vi "PC_PumpMeas.vi"() -> ()   [LabVIEW 2020]
doc: "PC Controller Main VI"
uses:
  TypeDefs/ApplyMultiplier.ctl
  TypeDefs/NI9205offset.ctl
  TypeDefs/RTdisplayTimedLoop_dt.ctl
  TypeDefs/ApplyOffset.ctl
  TypeDefs/NI9205multiplier.ctl
  TypeDefs/NI9208offset.ctl
  TypeDefs/NI9208multiplier.ctl
  Components/DisplayWaveform/DisplayWaveforms/DisplayWaveforms.lvclass
  C:/Program Files (x86)/National Instruments/LabVIEW 2020/vi.lib/JKI/JKI SMO/SMO/SMO.lvclass
  C:/Program Files (x86)/National Instruments/LabVIEW 2020/vi.lib/JKI/JKI SMO/SMO.UI/SMO.UI.lvclass
  Components/DisplayWaveform/DisplayWaveforms/Typedefs/Dependencies--Cluster.ctl
  RT Target/PumpMeasurement/TypeDefs/STMLoopState_enum.ctl
  <vilib>/JKI/JKI SMO/SMO/Typedefs/SMOState --Enum.ctl
  Components_global/Queues/InterProcessQueueCtl.ctl
  TypeDefs/ConfigCluster.ctl
  TypeDefs/GraphInfoCluster.ctl
  <vilib>/NI/STM/TCP/TCP Read Options.ctl
  TypeDefs/AIloopTimes.ctl
  <vilib>/NI/STM/TCP/Read Meta Data (TCP Ref).vi
  f38d6d6a-e512-492a-acdc-1d388213210b.vi
  78bd2656-12e6-4809-88cd-6a89556620fb.vi
  <vilib>/NI/STM/TCP/Get Connection Reference (TCP).vi
  <vilib>/NI/STM/TCP/Read Meta Data (TCP Clst).vi
  <vilib>/JDP Science/JSONtext/JSON text to Variant.vi
  <vilib>/JDP Science/JSONtext/Variant to JSON Text.vi
  <vilib>/NI/STM/TCP/Read Message (TCP).vi
  <vilib>/NI/STM/TCP/Write Message (TCP).vi
  <vilib>/JDP Science/JSONtext/LVClass Serializer/JSONtext LVClass Serializer.lvclass
  <vilib>/NI/STM/NI STM.lvlib
  <vilib>/JKI/JKI SMO/SMO/SMO.lvclass
  <vilib>/JKI/JKI SMO/SMO.UI/SMO.UI.lvclass
  Components_global/Queues/Queues.lvlib
  <vilib>/JDP Science/JSONtext/JSONtext.lvlib
panel:
  in  "Update Chart?":bool
  in  "Clear Chart":bool
  in  "Export":bool
  in  "Stop":bool
  out "Status":string
  in  "Tab Control":enum32{"Information"}(tab)
  in  "NI9208 Multiplier":T1
  in  "NI9208 Offset":T2={"NI9208 Offset"=[0.0, 0.0, 0.0, 0.0, 0.0]}
  in  "NI9205 Multiplier":T3
  in  "Apply Offset?":T4
  out "NI9208 loop time [ms]":dbl=10.0 caption="Numeric"
  in  "RT Display Reader Loop Time [ms]":T5=1000 caption="Numeric"
  in  "Load\nConfig":bool
  in  "Save\nConfig":bool
  in  "NI9205 Offset":T6={"NI9205 Offset"=[0.0, 0.0, 0.0, 0.0, 0.0, 0.0, 0.0, 0.0, 0.0, 0.0, 0.0, 0.0, 0.0, 0.0, 0.0]}
  out "# of display elements \nunpacked (row x col)":i32[](array[numeric]) caption="Numeric"
  out "NI9205 loop time [ms]":dbl caption="Numeric"
  in  "Apply Multiplier?":T7
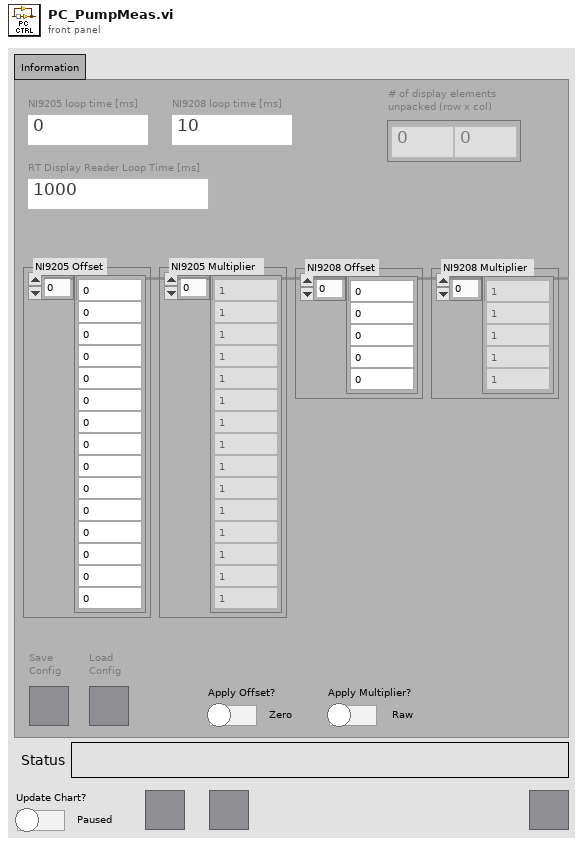
[diagram p1: front panel]
types:
  T1 = typedef "NI9208multiplier.ctl" = cluster{"NI9208 Multiplier":dbl[]}
  T2 = typedef "NI9208offset.ctl" = cluster{"NI9208 Offset":dbl[]}
  T3 = typedef "NI9205multiplier.ctl" = cluster{"NI9205 Multiplier":dbl[]}
  T4 = typedef "ApplyOffset.ctl" = bool
  T5 = typedef "RTdisplayTimedLoop_dt.ctl" = i64
  T6 = typedef "NI9205offset.ctl" = cluster{"NI9205 Offset":dbl[]}
  T7 = typedef "ApplyMultiplier.ctl" = bool
  T8 = typedef "STMLoopState_enum.ctl" = enum16{"Initialize", "Warm-up", "Run", "ShutDown"}
  T9 = typedef "DisplayWaveform.lvlib/DisplayWaveforms.lvclass/Dependencies--Cluster.ctl" = cluster{"New Value":refnum<user-event>}
  T10 = typedef "SMO.lvclass/Public Events.ctl" = cluster{"Error":refnum<user-event>, "State":refnum<user-event>, "Reserve State":refnum<user-event>}
  T11 = typedef "SMO.UI.lvclass/PublicEvents--Cluster.ctl" = cluster{"UI Hidden":refnum<user-event>, "UI State":refnum<user-event>}
  T12 = typedef "DisplayWaveform.lvlib/DisplayWaveforms.lvclass/PublicEvents--Cluster.ctl" = cluster{"Chart Cleared":refnum<user-event>, "Chart Exported":refnum<user-event>, "ChartParams Set":refnum<user-event>}
  T13 = typedef "NI STM.lvlib/TCP Connection Info.ctl" = cluster{"connection ID":refnum<k5>, "meta data":T14[]}
  T14 = typedef "NI STM.lvlib/MetaDataElement.ctl" = string
  T15 = typedef "Queues.lvlib/Queue Refs.ctl" = cluster{"InterProcessQueue":refnum<queue>}
  T16 = typedef "SMO.lvclass/SMOState --Enum.ctl" = enum16{"unknown", "Created", "Started", "Stopped"}
  T17 = enum32{"Invalid", "Standard", "Closed", "Hidden", "Minimized", "Maximized"}
  T18 = enum32{"invalid app kind", "Development System", "Run Time System", "Student Edition", "Embedded LabVIEW", "Evaluation", "Custom"}
  T19 = typedef "Queues.lvlib/InterProcessQueueCtl.ctl" = cluster{"Command":string, "Data":variant}
  T20 = typedef "ConfigCluster.ctl" = cluster{"RT Display Reader Loop Time [ms]":i64, "NI9205 Offset":T6, "NI9205 Multiplier":T3, "NI9208 Offset":T2, "NI9208 Multiplier":T1, "Apply Offset?":T4, "Apply Multiplier?":T7}
  T21 = enum16{"open", "replace", "create", "open or create", "replace or create", "replace or create with confirmation"}
  T22 = typedef "GraphInfoCluster.ctl" = cluster{"RT Display Reader Loop Time [ms]":T5, "NI9205 Offset":T6, "NI9205 Multiplier":T3, "NI9208 Offset":T2, "NI9208 Multiplier":T1}
  T23 = cluster{"Core":cluster{"Current VI Reference":refnum<vi>, "Close Panel on Exit?":bool}, "UI switch state":bool, "Export Folder Path":path}
  T24 = cluster{"Current VI Reference":refnum<vi>, "Close Panel on Exit?":bool}
  T25 = typedef "ChartParamsCluster.ctl" = cluster{"Chart ScaleMultipliers":cluster{"WF Xscale Multiplier":dbl, "WF Yscale Multiplier":dbl[]}, "NI9205 Offset":T6, "NI9205 Multipliers":T3, "NI9208 Offset":T2, "NI9208 Multiplier":T1}
  T26 = typedef "NI STM.lvlib/TCP Read Options.ctl" = cluster{"ignore timeout error":bool, "timeout ms (1000)":i32}
  T27 = typedef "AIloopTimes.ctl" = cluster{"NI 9205 loop time":dbl, "NI 9208 loop time":dbl}
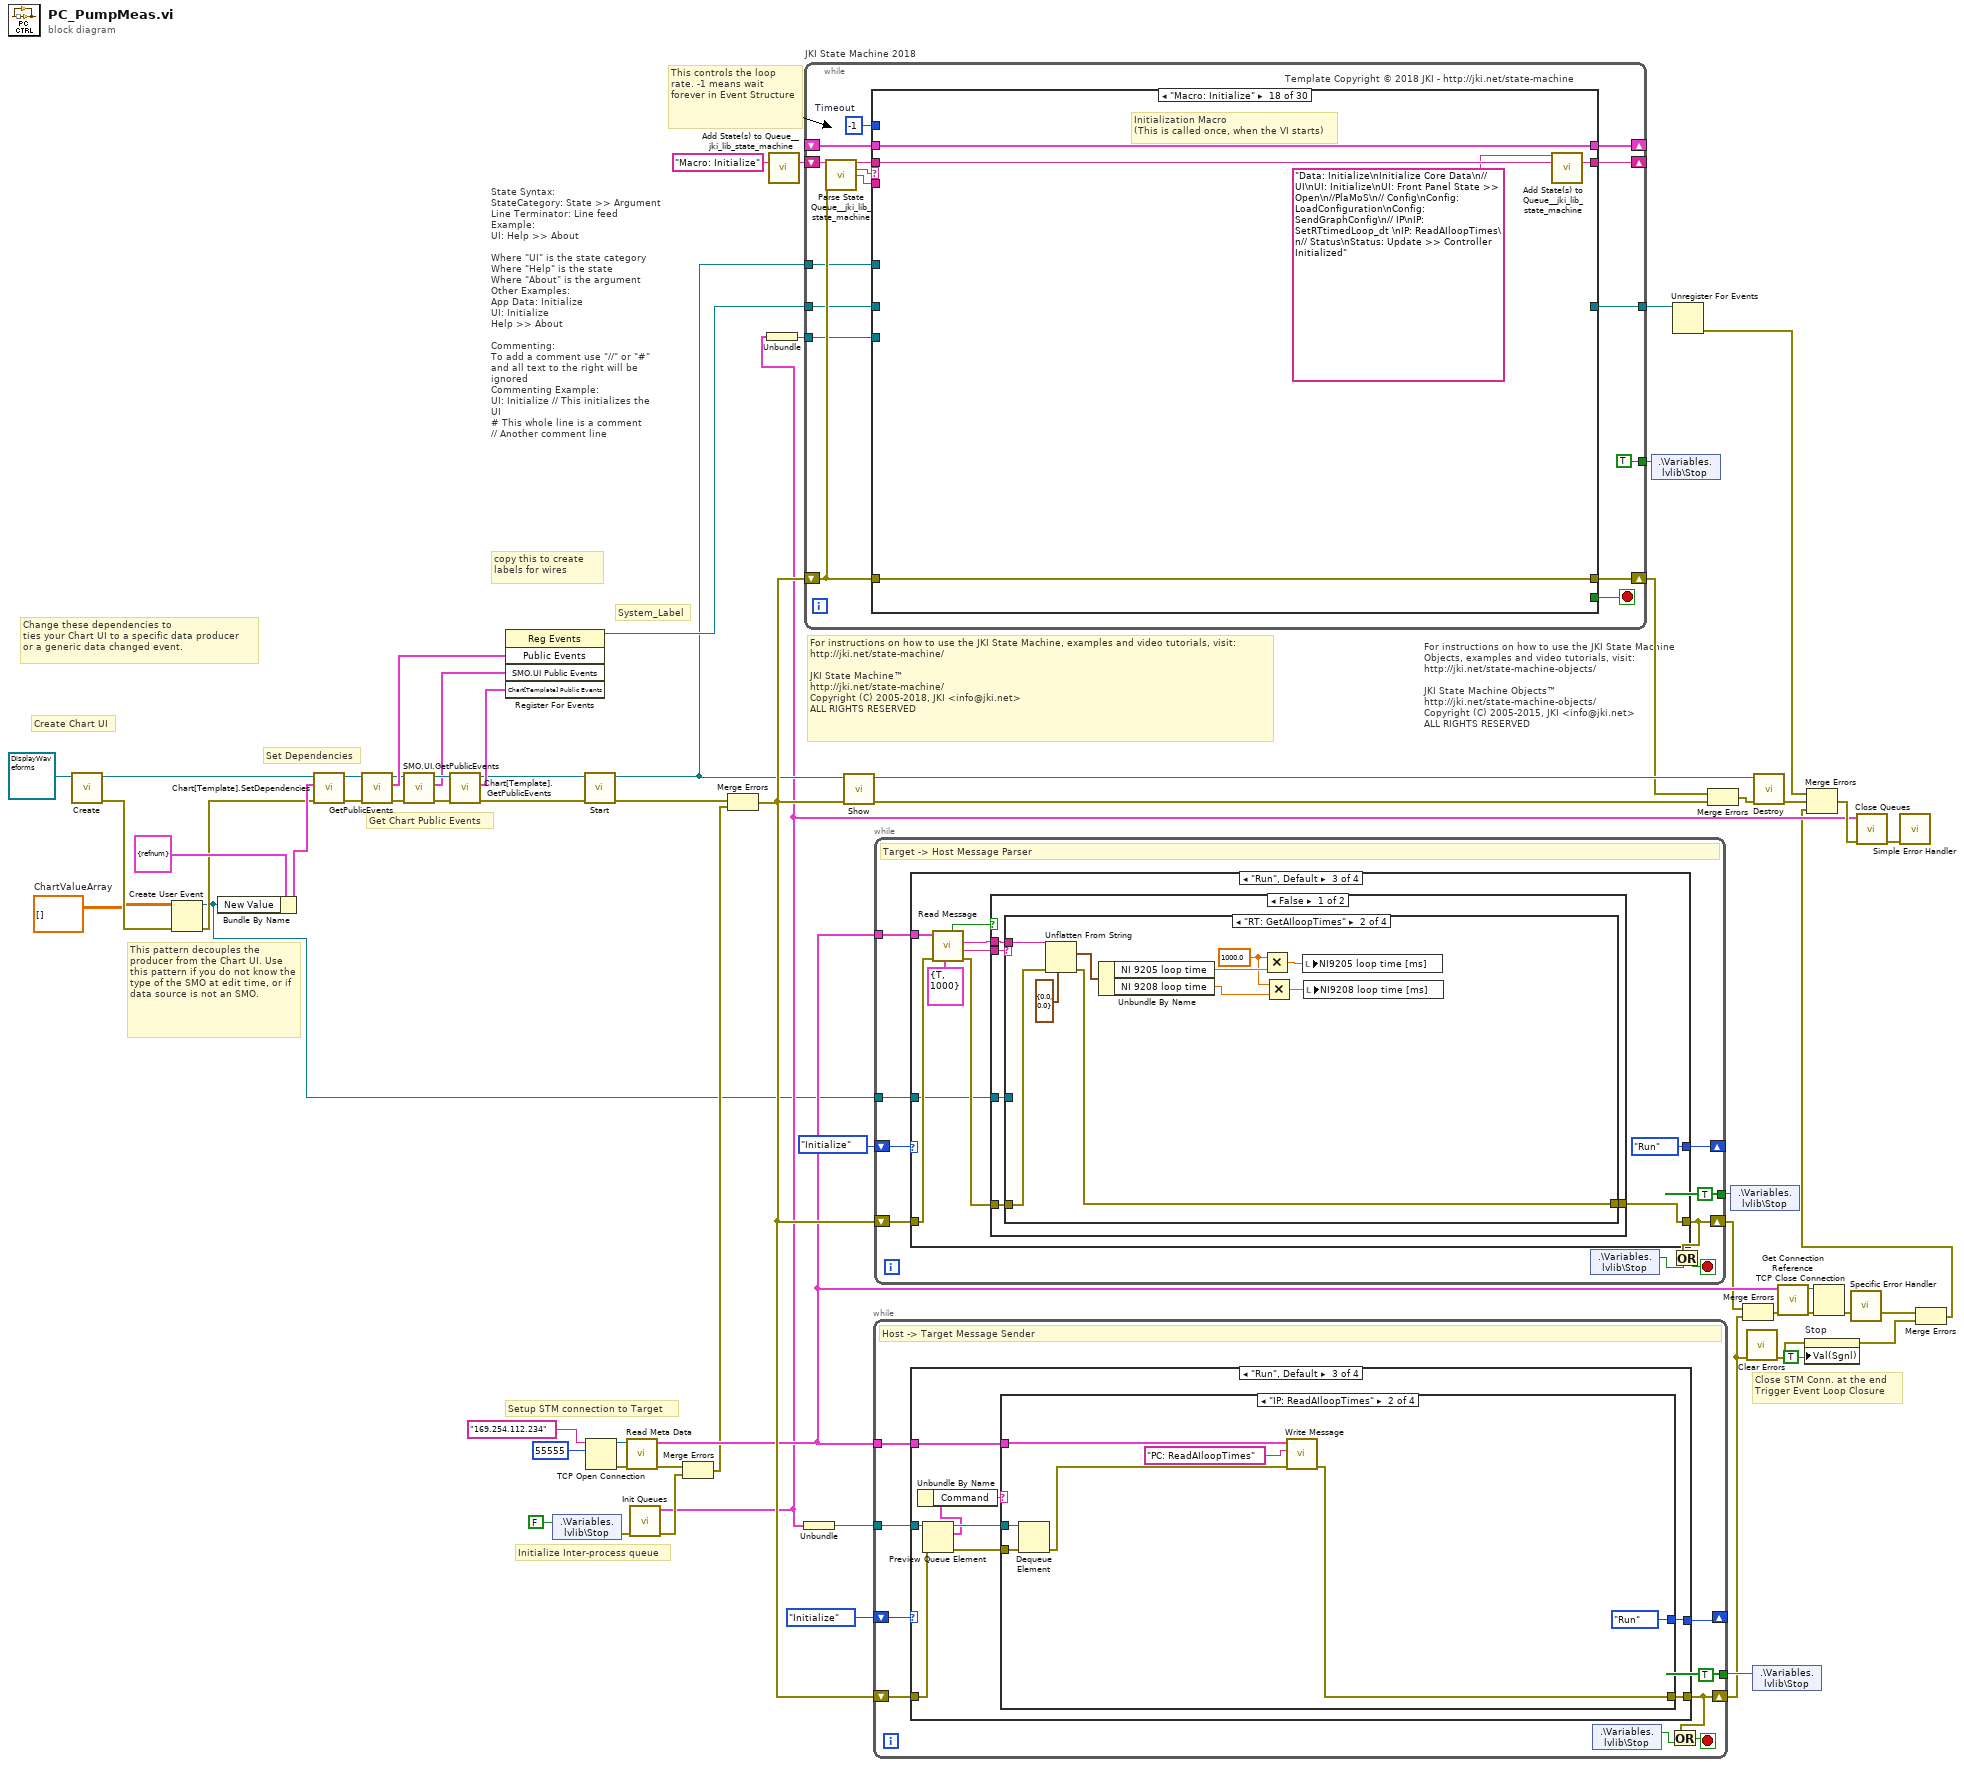
[diagram p0: block diagram]
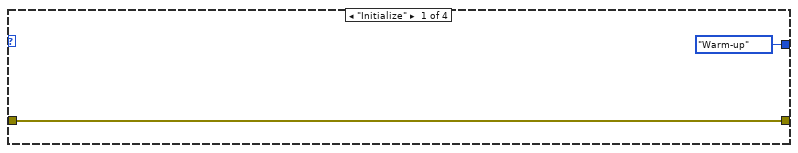
[diagram p2: hidden frame]
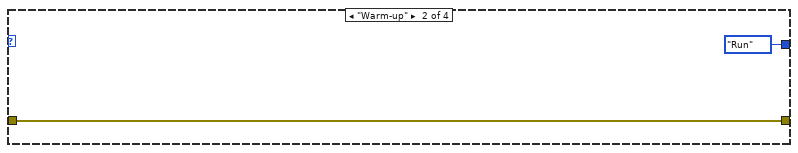
[diagram p3: hidden frame]
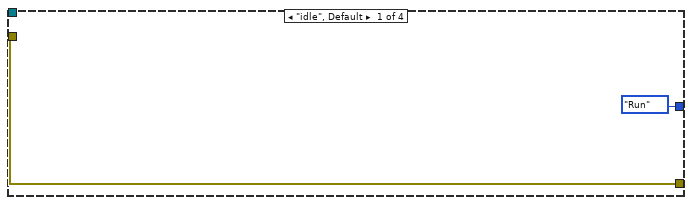
[diagram p4: hidden frame]
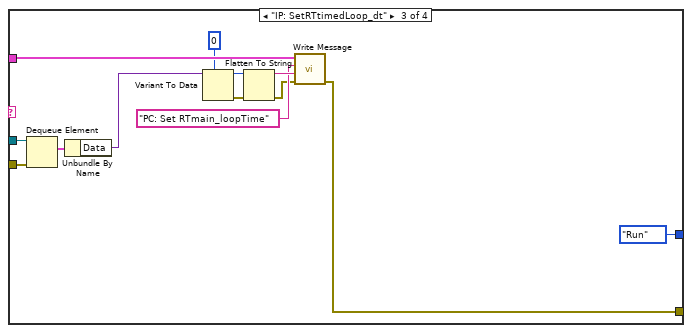
[diagram p5: hidden frame]
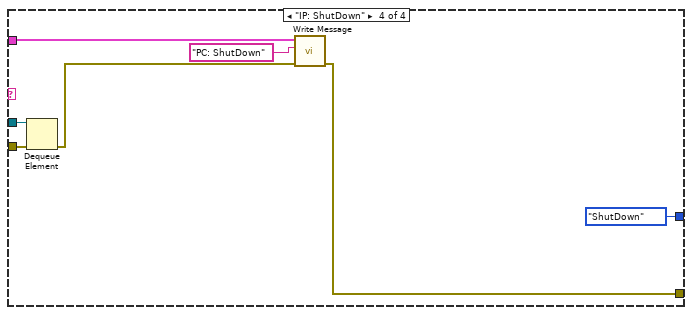
[diagram p6: hidden frame]
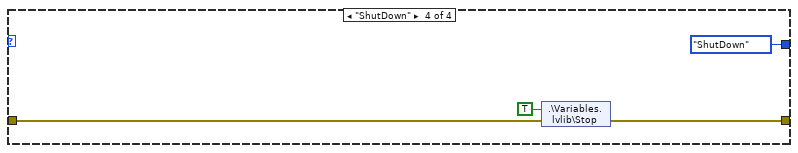
[diagram p7: hidden frame]
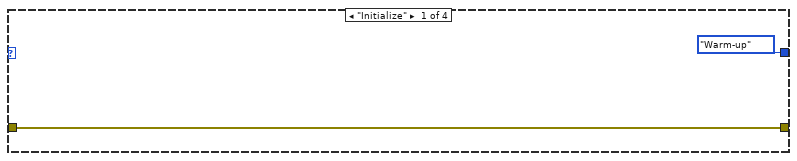
[diagram p8: hidden frame]
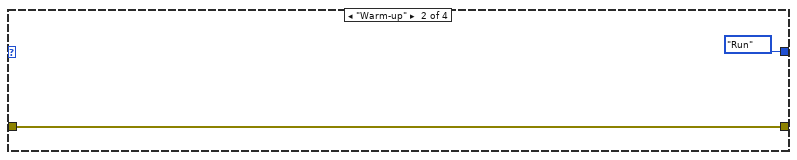
[diagram p9: hidden frame]
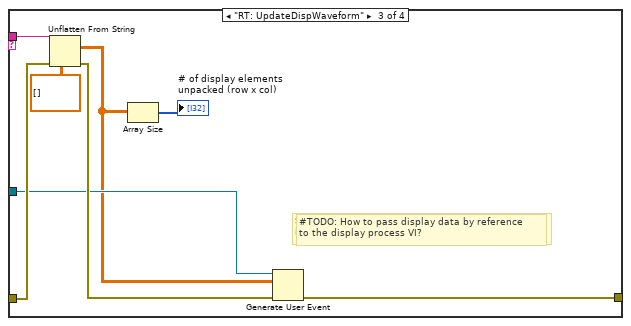
[diagram p11: hidden frame]
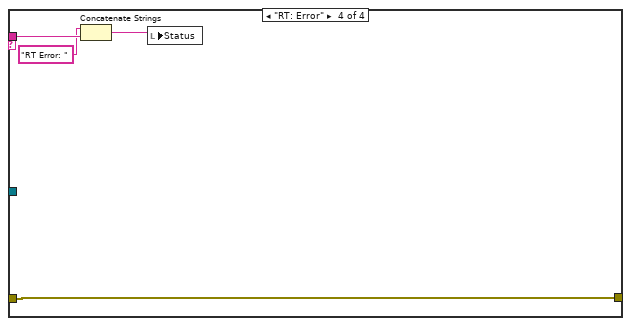
[diagram p12: hidden frame]
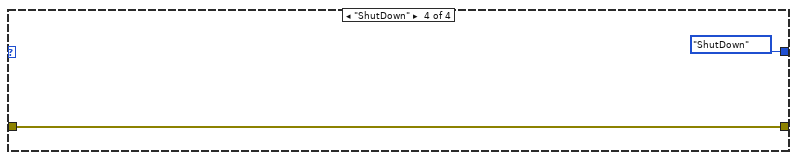
[diagram p14: hidden frame]
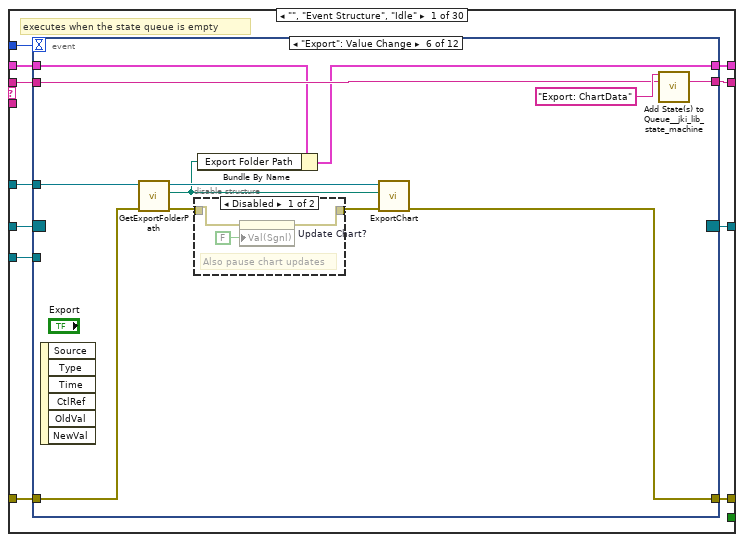
[diagram p15: hidden frame]
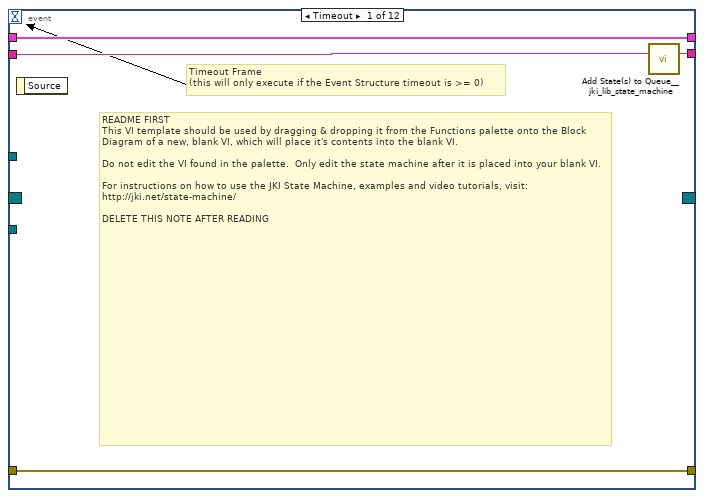
[diagram p16: hidden frame]
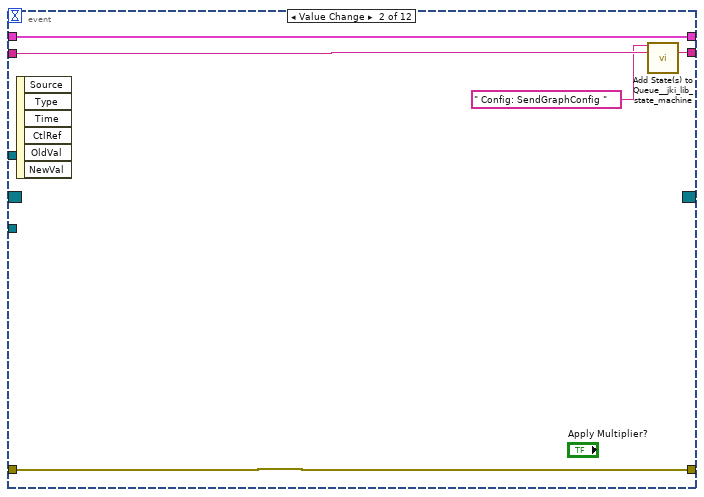
[diagram p17: hidden frame]
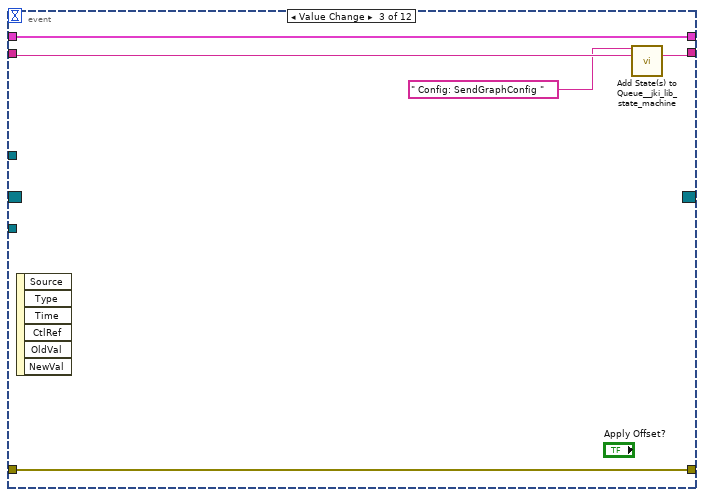
[diagram p18: hidden frame]
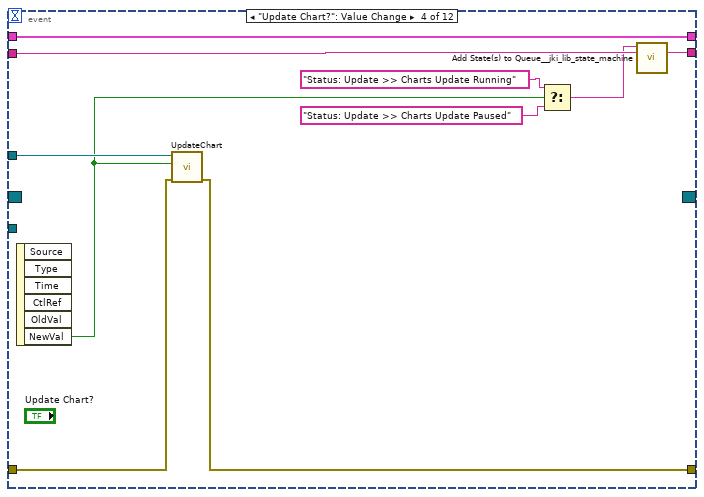
[diagram p19: hidden frame]
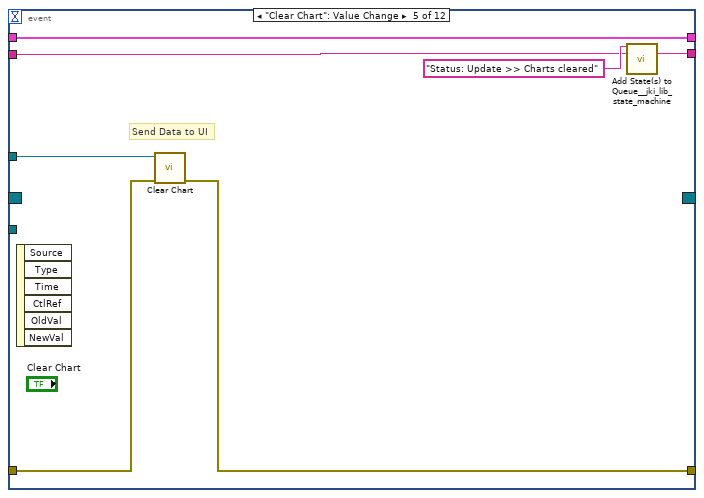
[diagram p20: hidden frame]
diagram:
  w9 = dbl[][] []  # ChartValueArray
  # "Close STM Conn. at the end\nTrigger Event Loop Closure"
  # "Setup STM connection to Target"
  # "Initialize Inter-process queue"
  # "This pattern decouples the producer from the Chart UI. Use this pattern if you do not know the type of the SMO at edit time, or if data source is not an SMO."
  # "For instructions on how to use the JKI State Machine, examples and video tutorials, visit:\nhttp://jki.net/state-machine/\n\nJKI State Machine™\nhttp://jki.net/state-machine/\nCopyright (C) 2005-2018, JKI <info@jki.net>\nALL RIGHTS RESERVED"
  # "State Syntax:\nStateCategory: State >> Argument\nLine Terminator: Line feed\nExample:\nUI: Help >> About\n\nWhere \"UI\" is the state category\nWhere \"Help\" is the state\nWhere \"About\" is the argument\nOther Examples:\nApp Data: Initialize\nUI: Initialize\nHelp >> About\n\nCommenting:\nTo add a comment use \"//\" or \"#\" and all text to the right will be ignored\nCommenting Example:\nUI: Initialize // This initializes the UI\n# This whole line is a comment\n// Another comment line"
  # "copy this to create labels for wires"
  # "This controls the loop rate. -1 means wait forever in Event Structure"
  # "System_Label"
  # "Set Dependencies"
  # "Create Chart UI"
  # "Change these dependencies to\nties your Chart UI to a specific data producer\nor a generic data changed event."
  # "For instructions on how to use the JKI State Machine Objects, examples and video tutorials, visit:\nhttp://jki.net/state-machine-objects/\n\nJKI State Machine Objects™\nhttp://jki.net/state-machine-objects/\nCopyright (C) 2005-2015, JKI <info@jki.net>\nALL RIGHTS RESERVED"
  # "Get Chart Public Events"
  n1 = call <vilib>:"Create.vi"("SMO"=refnum<class "DisplayWaveforms.lvclass"> refnum ("Chart[Template]")) -> ("error out"=w11:errorcluster, "SMO out"=w55:refnum<class "DisplayWaveforms.lvclass">)  [unwired: 8 in, 1 out]
  n2 = Create User Event(user event datatype=w9, error in=w11) -> (user event=w8:refnum<user-event>, error out=w10:errorcluster)
  n3 = Bundle By Name(cluster=T9 {"New Value"=refnum} ("Dependencies"), "New Value"=w8) -> (w53:T9)
  n4 = call "Chart[Template].SetDependencies.vi"("error in (no error)"=w10, "Dependencies"=w53, "DisplayWaveforms"=w55) -> ("error out"=w41:errorcluster, "DisplayWaveforms out"=w52:refnum<class "DisplayWaveforms.lvclass">)  [unwired: 7 in]
  n5 = call <vilib>:"GetPublicEvents.vi"("error in (no error)"=w41, "SMO"=w52) -> ("error out"=w47:errorcluster, "Public Events"=w51:T10, "SMO out"=w49:refnum<class "DisplayWaveforms.lvclass">)  [unwired: 7 in]
  n6 = call <vilib>:"SMO.UI.GetPublicEvents.vi"("error in (no error)"=w47, "SMO.UI"=w49) -> ("error out"=w46:errorcluster, "SMO.UI Public Events"=w45:T11, "SMO.UI out"=w48:refnum<class "DisplayWaveforms.lvclass">)  [unwired: 7 in]
  n7 = call "Chart[Template].GetPublicEvents.vi"("error in (no error)"=w46, "DisplayWaveforms"=w48) -> ("error out"=w42:errorcluster, "Chart[Template] Public Events"=w50:T12, "DisplayWaveforms out"=w43:refnum<class "DisplayWaveforms.lvclass">)  [unwired: 7 in]
  n8 = register-events(w51, w45, w50) -> (reference out=w44:refnum<event-registration>)  [unwired: 2 in, 1 out]
  n9 = shared-variable ".\\Variables.lvlib\\Stop"(FALSE ("Stop")) -> (error out=w32:errorcluster)  [unwired: 1 in]
  n10 = call <vilib>:"Start.vi"("error in (no error)"=w42, "SMO"=w43) -> ("error out"=w27:errorcluster, "SMO out"=w25:refnum<class "DisplayWaveforms.lvclass">)  [unwired: 8 in]
  n11 = TCP Open Connection(address="169.254.112.234" ("Target IP Address"), remote port or service name=u16 55555 ("remote port")) -> (connection ID=w63:refnum<k5>, error out=w62:errorcluster)  [unwired: 1 in, 2 out]
  n12 = call-poly <vilib>:"Read Meta Data.vi"("error in"=w62, "connection ID"=w63) -> ("error out"=w16:errorcluster, "connection info out"=w21:T13)  [unwired: 1 in, 7 out]
  n13 = call "Init Queues.vi"("error in (no error)"=w32) -> ("error out"=w15:errorcluster, "Queue Refs"=w12:T15)  [unwired: 9 in]
  n14 = Merge Errors(w16, w15) -> (w14:errorcluster)
  n15 = Merge Errors(w27, w14) -> (w26:errorcluster)
  n16 = Unbundle(w12) -> ("InterProcessQueue"=w13:refnum<queue>)
  n17 = call <vilib>:"Add State(s) to Queue__jki_lib_state_machine.vi"("State(s) in (\"\")"="Macro: Initialize") -> ("States Out"=w39:string)  [unwired: 14 in]
  n18 = Unbundle(w12) -> ("InterProcessQueue"=w28:refnum<queue>)
  n19 = while "JKI State Machine 2018" {
    shift-right: [w66] -> _
    shift-left: _ -> [w72]
    shift-right: [w74] -> _
    shift-left: w39 -> [w76]
    tunnel: w44 -> [w69]
    tunnel: w25 -> [w68]
    tunnel: [w67] -> w37
    tunnel: [TRUE ("Stop")] -> w35
    shift-right: [w75] -> w7
    shift-left: w26 -> [w70]
    tunnel: w13 -> [w64]
    stop <- w73 stop-if-true
    w71 = -1  # Timeout
    # "Template Copyright © 2018 JKI - http://jki.net/state-machine"
    n20 = call <vilib>:"Parse State Queue__jki_lib_state_machine.vi"("State Queue"=w76, "Error In (no error)"=w70) -> ("Remaining States"=w78:string, "Current State"=w79:string, "Arguments"=w77:string)  [unwired: 11 in]
    n21 = case shown="\"Macro: Initialize\"" w79 {
      selector: w79 -> [_ _ w188 _ _ _ _ _ _ _ _ _ _ _ _ _ _ _ _ _ _ _ _ _ _ _ _ _ _ _]
      tunnel: w78 -> [w90 w187 w192 w211 w213 w225 w229 w236 w242 w246 w254 w263 w274 w343 w352 w364 w368 w373 w390 w394 w423 w451 w474 w493 w502 w506 w511 w515 w519 w523]
      tunnel: w77 -> [_ _ _ _ _ _ _ _ _ _ _ w258 w268 _ _ _ _ _ _ _ _ w433 _ _ w494 _ _ _ _ _]
      tunnel: w72 -> [w88 w184 w190 w204 w217 w223 w226 _ w237 w243 w252 w261 w270 w340 w346 w362 w365 w370 w388 w391 w421 w432 w477 w490 w499 w503 w508 w512 w516 w520]
      tunnel: [w87 w185 w194 w208 errorcluster {"status"=FALSE, "code"=0, "source"=""} ("error out") w222 w227 w233 w238 w244 w247 w259 w271 w341 w344 w354 w366 w371 w375 w392 w408 w436 w469 w491 w500 w504 w509 w513 w517 w521] -> w75
      tunnel: w70 -> [w86 w185 w193 w208 w216 w222 w227 w233 w239 w244 w249 w260 w272 w341 w345 w355 w366 w371 w377 w392 w416 w437 w470 w491 w500 w504 w509 w513 w517 w521]
      tunnel: [w89 w186 w191 w210 w219 w224 w228 w235 w241 w245 w253 w262 w273 w342 w351 w363 w367 w372 w389 w393 w422 w450 w475 w492 w501 w505 w510 w514 w518 w522] -> w74
      tunnel: [_ _ _ _ _ TRUE _ _ _ _ _ _ _ _ _ _ _ _ _ _ _ _ _ _ _ _ _ _ _ _] -> w73
      tunnel: [w85 w184 w190 w209 w217 w223 w226 w234 w237 w243 w252 w261 w270 w340 w346 w362 w365 w370 w388 w391 w421 w432 w477 w490 w499 w503 w508 w512 w516 w520] -> w66
      tunnel: w71 -> [w84 _ _ _ _ _ _ _ _ _ _ _ _ _ _ _ _ _ _ _ _ _ _ _ _ _ _ _ _ _]
      tunnel: w69 -> [w83 _ _ _ _ w220 _ _ _ _ _ _ _ _ _ _ _ _ _ _ _ _ _ _ _ _ _ _ _ _]
      tunnel: w68 -> [w82 _ _ _ _ _ _ _ _ _ _ _ _ _ _ _ _ _ _ _ _ _ w473 _ _ _ _ _ _ _]
      tunnel: [w81 _ _ _ _ w220 _ _ _ _ _ _ _ _ _ _ _ _ _ _ _ _ _ _ _ _ _ _ _ _] -> w67
      tunnel: w64 -> [w80 _ _ _ _ _ _ _ _ _ _ _ _ _ w347 w356 _ _ w374 _ _ _ _ _ _ _ _ _ _ _]
      frame "", "Event Structure", "Idle" {
        # "executes when the state queue is empty"
        n22 = event shown="[5] \"Export\": Value Change" {
          selector: w83 -> [_ _ _ _ _ _ _ _ _ _ _ _]
          dyn-events: [_ _ _ _ _ _ _ _ _ _ _ _] -> w81
          timeout: w84 -> [_ _ _ _ _ _ _ _ _ _ _ _]
          tunnel: w90 -> [w94 w98 w103 w110 w116 w131 w140 w145 w158 w168 w172 w179]
          tunnel: [w93 w99 w104 w109 w115 w130 w141 w146 w157 w167 w171 w179] -> w89
          tunnel: w88 -> [w91 w95 w102 w111 w118 w126 w142 w147 w156 w166 w173 w180]
          tunnel: [w92 w96 w100 w112 w119 w133 w138 w143 w148 w159 w174 w181] -> w87
          tunnel: w86 -> [w92 w96 w100 w113 w120 w127 w138 w143 w151 w160 w174 w182]
          tunnel: [w91 w95 w102 w111 w118 w124 w142 w147 w156 w166 w173 w180] -> w85
          tunnel: w82 -> [_ _ _ w114 w121 w129 _ _ w152 w161 _ w183]
          tunnel: w80 -> [_ _ _ _ _ _ _ _ _ _ _ _]
          event Timeout {
            # "README FIRST\nThis VI template should be used by dragging & dropping it from the Functions palette onto the Block Diagram of a new, blank VI, which will place it's contents into the blank VI.\n\nDo not edit the VI found in the palette.  Only edit the state machine after it is placed into your blank VI.\n\nFor instructions on how to use the JKI State Machine, examples and video tutorials, visit:\nhttp://jki.net/state-machine/\n\nDELETE THIS NOTE AFTER READING"
            # "Timeout Frame\n(this will only execute if the Event Structure timeout is >= 0)"
            n23 = event-data() -> ()  [unwired: 1 in, 1 out]
            n24 = call <vilib>:"Add State(s) to Queue__jki_lib_state_machine.vi"("State(s) in (\"\")"=w94) -> ("States Out"=w93:string)  [unwired: 14 in]
          }
          event Value Change {
            n25 = event-data() -> ()  [unwired: 1 in, 6 out]
            n26 = call <vilib>:"Add State(s) to Queue__jki_lib_state_machine.vi"("State(s) in Front (\"\")"=" Config: SendGraphConfig " ("State(s) in Front (\"\")"), "State(s) in (\"\")"=w98) -> ("States Out"=w99:string)  [unwired: 13 in]
          }
          event Value Change {
            n27 = event-data() -> ()  [unwired: 1 in, 6 out]
            n28 = call <vilib>:"Add State(s) to Queue__jki_lib_state_machine.vi"("State(s) in Front (\"\")"=" Config: SendGraphConfig " ("State(s) in Front (\"\")"), "State(s) in (\"\")"=w103) -> ("States Out"=w104:string)  [unwired: 13 in]
          }
          event "Update Chart?": Value Change {
            n29 = event-data() -> ("NewVal"=w105:bool)  [unwired: 1 in, 5 out]
            n30 = call "UpdateChart.vi"("error in (no error)"=w113, "Update Chart?"=w105, "DisplayWaveforms"=w114) -> ("error out"=w112:errorcluster)  [unwired: 7 in, 1 out]
            n31 = Select(t="Status: Update >> Charts Update Running" ("State(s) in Front (\"\")"), s=w105, f="Status: Update >> Charts Update Paused" ("State(s) in Front (\"\")")) -> (s? t:f=w106:string)
            n32 = call <vilib>:"Add State(s) to Queue__jki_lib_state_machine.vi"("State(s) in Front (\"\")"=w106, "State(s) in (\"\")"=w110) -> ("States Out"=w109:string)  [unwired: 13 in]
          }
          event "Clear Chart": Value Change {
            # "Send Data to UI"
            n33 = event-data() -> ()  [unwired: 1 in, 6 out]
            n34 = call "Clear Chart.vi"("error in (no error)"=w120, "DisplayWaveforms"=w121) -> ("error out"=w119:errorcluster)  [unwired: 8 in, 1 out]
            n35 = call <vilib>:"Add State(s) to Queue__jki_lib_state_machine.vi"("State(s) in Front (\"\")"="Status: Update >> Charts cleared" ("State(s) in Front (\"\")"), "State(s) in (\"\")"=w116) -> ("States Out"=w115:string)  [unwired: 13 in]
          }
          event "Export": Value Change {
            n36 = event-data() -> ()  [unwired: 1 in, 6 out]
            n37 = call "GetExportFolderPath.vi"("error in (no error)"=w127, "DisplayWaveforms"=w129) -> ("error out"=w123:errorcluster, "Export File Folder"=w125:path, "DisplayWaveforms out"=w128:refnum<class "DisplayWaveforms.lvclass">)  [unwired: 7 in]
            n38 = disable-structure shown="Disabled" {
              disable-tunnel: w123 -> [w135 w137]
              disable-tunnel: [w134 w137] -> w122
              frame Disabled {
                # "Also pause chart updates"
                n39 = property on="Update Chart?" class="Bool (strict)"(error in=w135, "Val(Sgnl)"=FALSE ("Value (Signaling)")) -> (error out=w134:errorcluster)  [unwired: 1 in, 1 out]
              }
              frame Enabled {
              }
            }
            n40 = Bundle By Name(cluster=w126, "Export Folder Path"=w125) -> (w124:T23)
            n41 = call "ExportChart.vi"("error in (no error)"=w122, "Export File Folder"=w125, "DisplayWaveforms"=w128) -> ("error out"=w133:errorcluster)  [unwired: 7 in, 1 out]
            n42 = call <vilib>:"Add State(s) to Queue__jki_lib_state_machine.vi"("State(s) in Front (\"\")"="Export: ChartData" ("State(s) in Front (\"\")"), "State(s) in (\"\")"=w131) -> ("States Out"=w130:string)  [unwired: 13 in]
          }
          event "Save\nConfig": Value Change {
            n43 = event-data() -> ()  [unwired: 1 in, 6 out]
            n44 = call <vilib>:"Add State(s) to Queue__jki_lib_state_machine.vi"("State(s) in Front (\"\")"="Config: SaveConfiguration", "State(s) in (\"\")"=w140) -> ("States Out"=w141:string)  [unwired: 13 in]
          }
          event "Load\nConfig": Value Change {
            # "LoadConfiguration file and set zero accordingly"
            n45 = event-data() -> ()  [unwired: 1 in, 6 out]
            n46 = call <vilib>:"Add State(s) to Queue__jki_lib_state_machine.vi"("State(s) in Front (\"\")"="Config: LoadConfiguration", "State(s) in (\"\")"=w145) -> ("States Out"=w146:string)  [unwired: 13 in]
          }
          event "Stop": Value Change {
            # "Stop Communication Process"
            # "Hide UI"
            # "Stop SMO if Stop was pressed"
            # "Exit Button Value Change (pressed) Event\n(this executes Macro: Exit to terminate the VI)"
            n47 = event-data() -> ()  [unwired: 1 in, 6 out]
            n48 = call <vilib>:"Hide.vi"("error in (no error)"=w151, "SMO.UI"=w152) -> ("error out"=w154:errorcluster, "SMO.UI out"=w153:refnum<class "DisplayWaveforms.lvclass">)  [unwired: 8 in]
            n49 = call <vilib>:"Stop.vi"("error in (no error)"=w154, "SMO"=w153) -> ("error out"=w149:errorcluster)  [unwired: 8 in, 1 out]
            n50 = property on="Stop" class="Bool (strict)"(error in=w149, "Value"=FALSE ("Stop")) -> (error out=w148:errorcluster)  [unwired: 1 in, 1 out]
            n51 = call <vilib>:"Add State(s) to Queue__jki_lib_state_machine.vi"("State(s) in Front (\"\")"="Macro: Exit", "State(s) in (\"\")"=w158) -> ("States Out"=w157:string)  [unwired: 13 in]
          }
          event Panel Close? {
            # "Stop SMO if Panel Closed"
            # "Discard the event because we'll close the front panel ourselves in Macro: Exit"
            # "Close Panel button (pressed) Event\n(this executes Macro: Exit to terminate the VI)"
            n52 = event-data() -> ()  [unwired: 1 in, 1 out]
            n53 = call <vilib>:"Hide.vi"("error in (no error)"=w160, "SMO.UI"=w161) -> ("error out"=w162:errorcluster, "SMO.UI out"=w163:refnum<class "DisplayWaveforms.lvclass">)  [unwired: 8 in]
            n54 = call <vilib>:"Stop.vi"("error in (no error)"=w162, "SMO"=w163) -> ("error out"=w159:errorcluster)  [unwired: 8 in, 1 out]
            n55 = event-data("Discard?"=TRUE) -> ()  [unwired: 1 in, 1 out]
            n56 = call <vilib>:"Add State(s) to Queue__jki_lib_state_machine.vi"("State(s) in Front (\"\")"="Macro: Exit", "State(s) in (\"\")"=w168) -> ("States Out"=w167:string)  [unwired: 13 in]
          }
          event User Event {
            n57 = event-data() -> ("SMO State"=w175:T16)  [unwired: 1 in, 4 out]
            n58 = Equal?(x=SMOState_--Enum."Stopped", y=w175) -> (x = y?=w170:bool)
            n59 = case shown="False" w170 {
              tunnel: ["Idle" "Macro: Exit"] -> w169
              frame False {
              }
              frame True {
              }
            }
            n60 = call <vilib>:"Add State(s) to Queue__jki_lib_state_machine.vi"("State(s) in Front (\"\")"=w169, "State(s) in (\"\")"=w172) -> ("States Out"=w171:string)  [unwired: 13 in]
          }
          event User Event {
            # "Stop SMO if UI Closed"
            n61 = event-data() -> ()  [unwired: 1 in, 5 out]
            n62 = call <vilib>:"Stop.vi"("error in (no error)"=w182, "SMO"=w183) -> ("error out"=w181:errorcluster)  [unwired: 8 in, 1 out]
          }
        }
      }
      frame "---------- Core ----------" {
        # "Do not put any code in this frame.\n(it is a separator no-op)"
        n63 = call <vilib>:"Add State(s) to Queue__jki_lib_state_machine.vi"("State(s) in (\"\")"=w187) -> ("States Out"=w186:string)  [unwired: 14 in]
      }
      frame Default {
        w197 = 42 items=["No error", "Argument error", "Memory is full", "Out of zone", "End of file", "File already open", "Generic file I/O error", "File not found", "File permission error", "Disk is full", "Duplicate path", "Too many files open", "System feature not enabled", "Resource file not found", "Cannot add resource", "Resource not found", "Image not found", "Image memory error", "Pen does not exist", "Config type invalid", "Config token not found", "Config parse error", "Config memory error", "Bad external code format", "Bad external code offset", "External code not present", "Null window", "Destroy window error", "Null menu", "Print aborted", "Bad print record", "Print driver error", "Windows error during printing", "Memory error during printing", "Print dialog error", "Generic print error", "Invalid device refnum", "Device not found", "Device parameter error", "Device unit error", "Cannot open device", "Device call aborted", "Generic error", "Cancelled by user", "Object ID too low", "Object ID too high", "Object not in heap", "Unknown heap", "Unknown object (invalid DefProc)", "Unknown object (DefProc not in table)", "Message out of range", "Invalid (null) method", "Unknown message", "Manager call not supported", "Bad address", "Network operation in progress", "Network operation timed out", "Connection is busy", "Network attribute not supported", "Network error", "Address in use", "System out of memory", "Connection aborted", "Connection refused", "Not connected", "Already connected", "Connection closed", "Initialization error (interapplication manager)", "Bad occurrence", "Wait on unbound occurrence handler", "Occurrence queue overflow", "Datalog type conflict", "Unused", "Unrecognized type (interapplication manager)", "Memory corrupt", "Failed to make temporary DLL", "Old CIN version", "Drag socket not found", "Failed to load drop-object", "Failed to register OLE object", "Failed to release OLE object", "Format specifier type mismatch", "Unknown format specifier", "Too few format specifiers", "Too many format specifiers", "Scan failed", "Newer CIN version", "Error converting to variant", "Runtime menu error", "Password tampered", "Variant attribute not found", "Incompatible variant data type", "Event data is not available", "Event Store is not present", "Occurrence is not found", "Event Queue is not created", "Event info is not available", "Refnum passed is NULL", "Error retrieving Class GUID", "Error retrieving CoClass GUID", "Error retrieving TypeLib GUID.", "Bad built application magic bytes.", "Specific driver is different from the specific driver associated with the Logical Name.", "There is no session opened to the class driver.", "Max Error", "MAX - Error with config objects", "MAX - Error loading configuration", "MAX - Group not supported"]
        # "Current State"
        # "Do not delete, rename, or modify this frame.\n(this is used to capture unhandled states and typos)"
        # "Handle mistyped state name (developer tool)"
        n64 = Format Into String(format string="Software Exception: Unhandled State \"%s\"." ("message"), error in=w193, w188) -> (resulting string=w196:string, error out=w195:errorcluster)  [unwired: 1 in]
        n65 = call <vilib>:"Error Cluster From Error Code.vi"("show call chain? (False)"=TRUE, "error in (no error)"=w195, "error message (\"\")"=w196, "error code (0)"=w197) -> ("error out"=w194:errorcluster)  [unwired: 5 in]
        n66 = call <vilib>:"Add State(s) to Queue__jki_lib_state_machine.vi"("State(s) in (\"\")"=w192) -> ("States Out"=w191:string)  [unwired: 14 in]
      }
      frame "Initialize Core Data" {
        # "Do not delete, rename, or modify this frame.\n(this is used to determine panel behavior on exit)"
        # "originally closed?"
        # "exe?"
        # "If panel starts closed or is an EXE, then close it when we exit"
        n67 = property class="VI"() -> ("FP.State"=w201:T17)  [unwired: 2 in, 2 out]
        n68 = property class="App"() -> ("App.Kind"=w207:T18)  [unwired: 2 in, 2 out]
        n69 = control-ref of="Current VI Reference"() -> (w202:refnum<vi>)
        n70 = Equal?(x=w201, y=T17."Closed" ("Front Panel Window:State")) -> (x = y?=w199:bool)
        n71 = Equal?(x=w207, y=T18."Run Time System" ("Application:Kind")) -> (x = y?=w205:bool)
        n72 = Or(x=w199, y=w205) -> (x .or. y?=w203:bool)
        n73 = Bundle By Name(cluster=w204, "Core.Current VI Reference"=w202, "Core.Close Panel on Exit?"=w203) -> (w209:T23)
        n74 = call <vilib>:"Add State(s) to Queue__jki_lib_state_machine.vi"("State(s) in (\"\")"=w211) -> ("States Out"=w210:string)  [unwired: 14 in]
      }
      frame "Error Handler" {
        # "Unhandled Error -- Display it"
        # "Handle any errors here.\nYou can also output any states to clean-up after errors occur"
        # "Clear error"
        n75 = Unbundle By Name(w216) -> ("source"=w214:string)
        n76 = call <vilib>:"General Error Handler.vi"("error in (no error)"=w216) -> ()  [unwired: 10 in, 5 out]
        n77 = Concatenate Strings("/*Post Error States\nStatus: Update >> PC Error: ", w214) -> (w212:string)
        n78 = call <vilib>:"Add State(s) to Queue__jki_lib_state_machine.vi"("State(s) in (\"\")"=w213, "State(s) at Back (\"\")"=w212) -> ("States Out"=w219:string)  [unwired: 13 in]
      }
      frame "Exit" {
        # "Do not put any code in this frame.\n(No errors that occur here will be handled.)"
        n79 = call <vilib>:"Add State(s) to Queue__jki_lib_state_machine.vi"("State(s) in (\"\")"=w225) -> ("States Out"=w224:string)  [unwired: 14 in]
      }
      frame "---------- Data ----------" {
        # "Do not put any code in this frame.\n(It is a separator no-op. You can make a copy of this frame to create a new Data frame)"
        n80 = call <vilib>:"Add State(s) to Queue__jki_lib_state_machine.vi"("State(s) in (\"\")"=w229) -> ("States Out"=w228:string)  [unwired: 14 in]
      }
      frame "Data: Initialize" {
        w230 = path ""  # Export Folder Path
        w231 = T24 {"Current VI Reference"=refnum, "Close Panel on Exit?"=FALSE}  # Core
        w232 = FALSE  # UI switch state
        # "Common Booelan for\nstoring state of any \nUI switch"
        # "Common Booelan for\nstoring state of any \nUI switch"
        # "do not delete - used by framework"
        # "Expand Bundle to add new data elements to shift register data."
        # "Add new data here."
        # "Data names and types of shift register data are defined by this bundle."
        # "Initialize the shift-register data, here.\n(data names are defined by what you wire into the bundle function)"
        n81 = Bundle("Core"=w231, "UI switch state"=w232, "Export Folder Path"=w230) -> (w234:T23)  [unwired: 1 in]
        n82 = call <vilib>:"Add State(s) to Queue__jki_lib_state_machine.vi"("State(s) in (\"\")"=w236) -> ("States Out"=w235:string)  [unwired: 14 in]
      }
      frame "Data: Cleanup" {
        # "Cleanup any data and references, here.\n(this is called automatically, by the Macro: Exit)"
        n83 = Unbundle By Name(w237) -> ("Core.Current VI Reference"=w240:refnum<vi>)
        n84 = Close Reference(reference=w240, error in (no error)=w239) -> (error out=w238:errorcluster)
        n85 = call <vilib>:"Add State(s) to Queue__jki_lib_state_machine.vi"("State(s) in (\"\")"=w242) -> ("States Out"=w241:string)  [unwired: 14 in]
      }
      frame "---------- UI ----------" {
        # "Do not put any code in this frame.\n(It is a separator no-op. You can make a copy of this frame to create a new UI frame)"
        n86 = call <vilib>:"Add State(s) to Queue__jki_lib_state_machine.vi"("State(s) in (\"\")"=w246) -> ("States Out"=w245:string)  [unwired: 14 in]
      }
      frame "UI: Initialize" {
        # "Initialize the User Interface, here.\n(this is called automatically, by the Macro: Init)"
        n87 = disable-structure shown="Enabled" {
          disable-tunnel: w249 -> [w256 _]
          disable-tunnel: [w255 _] -> w248
          frame Enabled {
            # "Reset All front panel controls"
            n88 = control-ref of="This VI"() -> (w257:refnum<vi>)
            n89 = invoke class="VI" method="Default Vals.Reinit All"(reference=w257, error in=w256) -> (error out=w255:errorcluster)  [unwired: 1 in, 2 out]
          }
          frame Disabled {
          }
        }
        n90 = property on="Update Chart?" class="Bool (strict)"(error in=w248, "Val(Sgnl)"=TRUE ("Value (Signaling)")) -> (error out=w247:errorcluster)  [unwired: 1 in, 1 out]
        n91 = call <vilib>:"Add State(s) to Queue__jki_lib_state_machine.vi"("State(s) in Front (\"\")"="Status: Update >> UI Initialized" ("State(s) in Front (\"\")"), "State(s) in (\"\")"=w254) -> ("States Out"=w253:string)  [unwired: 13 in]
      }
      frame "UI: Cursor Set" {
        # "Argument"
        # "Set and Unset Cursor Busy.\n(Usage: \"UI: Cursor Set >> Busy|Idle\")"
        n92 = case shown="\"Idle\", Default" w258 {
          tunnel: w260 -> [w265 w267]
          tunnel: [w264 w266] -> w259
          frame "Idle", Default {
            n93 = call <vilib>:"Unset Busy.vi"("error in (no error)"=w265) -> ("error out"=w264:errorcluster)  [unwired: 10 in]
          }
          frame "Busy" {
            n94 = call <vilib>:"Set Busy.vi"("error in (no error)"=w267) -> ("error out"=w266:errorcluster)  [unwired: 9 in, 1 out]
          }
        }
        n95 = call <vilib>:"Add State(s) to Queue__jki_lib_state_machine.vi"("State(s) in (\"\")"=w263) -> ("States Out"=w262:string)  [unwired: 14 in]
      }
      frame "UI: Front Panel State" {
        # "Argument"
        # "Set Front Panel Open or Closed\n(Usage: \"UI: Front Panel State >> Open|Close\")"
        n96 = Unbundle By Name(w270) -> ("Core.Current VI Reference"=w269:refnum<vi>)
        n97 = case shown="\"Open\", \"Standard\", Default" w268 {
          tunnel: w272 -> [w280 w295 w306 w319 w332]
          tunnel: [w282 w296 w308 w321 w334] -> w271
          tunnel: w269 -> [w281 w293 w307 w320 w333]
          frame "Open", "Standard", Default {
            w275 = T17."Standard" ("State")
            n98 = property class="VI"(reference=w281, error in=w280) -> (reference out=w278:refnum<vi>, error out=w279:errorcluster, "FP.State"=w277:T17)
            n99 = Not Equal?(x=w277, y=w275) -> (x != y?=w276:bool)
            n100 = case shown="False" w276 {
              tunnel: [w286 w288] -> w282
              tunnel: w279 -> [w285 w288]
              tunnel: w278 -> [w284 _]
              tunnel: w275 -> [w283 _]
              frame True {
                n101 = invoke class="VI" method="FP.Open"(reference=w284, error in=w285, "Activate"=TRUE, "State"=w283) -> (error out=w286:errorcluster)  [unwired: 1 in, 4 out]
              }
              frame False {
              }
            }
          }
          frame "Close", "Closed" {
            n102 = property class="VI"(reference=w293, error in=w295) -> (reference out=w292:refnum<vi>, error out=w294:errorcluster, "FP.State"=w290:T17)
            n103 = Not Equal?(x=w290, y=T17."Closed" ("Front Panel Window:State")) -> (x != y?=w289:bool)
            n104 = case shown="True" w289 {
              tunnel: [w297 w300] -> w296
              tunnel: w294 -> [w297 w299]
              tunnel: w292 -> [_ w298]
              frame False {
              }
              frame True {
                n105 = invoke class="VI" method="FP.Close"(reference=w298, error in=w299) -> (error out=w300:errorcluster)  [unwired: 1 in, 2 out]
              }
            }
          }
          frame "Hidden", "Hide" {
            w301 = T17."Hidden" ("State")
            n106 = property class="VI"(reference=w307, error in=w306) -> (reference out=w304:refnum<vi>, error out=w305:errorcluster, "FP.State"=w303:T17)
            n107 = Not Equal?(x=w303, y=w301) -> (x != y?=w302:bool)
            n108 = case shown="True" w302 {
              tunnel: [w312 w313] -> w308
              tunnel: w305 -> [w311 w313]
              tunnel: w304 -> [w310 _]
              tunnel: w301 -> [w309 _]
              frame True {
                n109 = invoke class="VI" method="FP.Open"(reference=w310, error in=w311, "State"=w309) -> (error out=w312:errorcluster)  [unwired: 2 in, 4 out]
              }
              frame False {
              }
            }
          }
          frame "Minimize", "Minimized" {
            w314 = T17."Minimized" ("State")
            n110 = property class="VI"(reference=w320, error in=w319) -> (reference out=w317:refnum<vi>, error out=w318:errorcluster, "FP.State"=w316:T17)
            n111 = Not Equal?(x=w316, y=w314) -> (x != y?=w315:bool)
            n112 = case shown="True" w315 {
              tunnel: [w325 w326] -> w321
              tunnel: w318 -> [w324 w326]
              tunnel: w317 -> [w323 _]
              tunnel: w314 -> [w322 _]
              frame True {
                n113 = invoke class="VI" method="FP.Open"(reference=w323, error in=w324, "State"=w322) -> (error out=w325:errorcluster)  [unwired: 2 in, 4 out]
              }
              frame False {
              }
            }
          }
          frame "Maximize", "Maximized" {
            w327 = T17."Maximized" ("State")
            n114 = property class="VI"(reference=w333, error in=w332) -> (reference out=w330:refnum<vi>, error out=w331:errorcluster, "FP.State"=w329:T17)
            n115 = Not Equal?(x=w329, y=w327) -> (x != y?=w328:bool)
            n116 = case shown="True" w328 {
              tunnel: [w338 w339] -> w334
              tunnel: w331 -> [w337 w339]
              tunnel: w330 -> [w336 _]
              tunnel: w327 -> [w335 _]
              frame True {
                n117 = invoke class="VI" method="FP.Open"(reference=w336, error in=w337, "State"=w335) -> (error out=w338:errorcluster)  [unwired: 2 in, 4 out]
              }
              frame False {
              }
            }
          }
        }
        n118 = call <vilib>:"Add State(s) to Queue__jki_lib_state_machine.vi"("State(s) in (\"\")"=w274) -> ("States Out"=w273:string)  [unwired: 14 in]
      }
      frame "---------- IP ----------" {
        # "Code for inter-process communication \nUse this to send messages via STM to RT target"
        # "Do not put any code in this frame.\n(It is a separator no-op. You can make a copy of this frame to create a new UI frame)"
        n119 = call <vilib>:"Add State(s) to Queue__jki_lib_state_machine.vi"("State(s) in (\"\")"=w343) -> ("States Out"=w342:string)  [unwired: 14 in]
      }
      frame "IP: ReadAIloopTimes" {
        # "Do not put any code in this frame.\n(It is a separator no-op. You can make a copy of this frame to create a new UI frame)"
        n120 = Bundle By Name(cluster=T19 {"Command"="", "Data"=variant} ("InterProcessQueue"), "Command"="IP: ReadAIloopTimes") -> (w349:T19)
        n121 = Enqueue Element(queue=w347, element=w349, error in (no error)=w345) -> (error out=w344:errorcluster)  [unwired: 1 in, 2 out]
        n122 = call <vilib>:"Add State(s) to Queue__jki_lib_state_machine.vi"("State(s) in (\"\")"=w352) -> ("States Out"=w351:string)  [unwired: 14 in]
      }
      frame "IP: SetRTtimedLoop_dt" {
        # "During Initialization, Set RT Display Timed Loop Rate"
        # "Do not put any code in this frame.\n(It is a separator no-op. You can make a copy of this frame to create a new UI frame)"
        n123 = local read "RT Display Reader Loop Time [ms]"() -> (w353:T5)
        n124 = To Quad Integer(1:w353) -> (0:w357:T5)
        n125 = To Variant(anything=w357) -> (Variant=w358:variant)
        n126 = Bundle By Name(cluster=T19 {"Command"="", "Data"=variant} ("InterProcessQueue"), "Command"="IP: SetRTtimedLoop_dt", "Data"=w358) -> (w360:T19)
        n127 = Enqueue Element(queue=w356, element=w360, error in (no error)=w355) -> (error out=w354:errorcluster)  [unwired: 1 in, 2 out]
        n128 = call <vilib>:"Add State(s) to Queue__jki_lib_state_machine.vi"("State(s) in (\"\")"=w364) -> ("States Out"=w363:string)  [unwired: 14 in]
      }
      frame "---------- Macro ----------" {
        # "Do not put any code in this frame.\n(It is a separator no-op. You can make a copy of this frame to create a new Macro frame)"
        n129 = call <vilib>:"Add State(s) to Queue__jki_lib_state_machine.vi"("State(s) in (\"\")"=w368) -> ("States Out"=w367:string)  [unwired: 14 in]
      }
      frame "Macro: Initialize" {
        # "Initialization Macro\n(This is called once, when the VI starts)"
        n130 = call <vilib>:"Add State(s) to Queue__jki_lib_state_machine.vi"("State(s) in Front (\"\")"="Data: Initialize\nInitialize Core Data\n// UI\nUI: Initialize\nUI: Front Panel State >> Open\n//PlaMoS\n// Config\nConfig: LoadConfiguration\nConfig: SendGraphConfig\n// IP\nIP: SetRTtimedLoop_dt \nIP: ReadAIloopTimes\n// Status\nStatus: Update >> Controller Initialized", "State(s) in (\"\")"=w373) -> ("States Out"=w372:string)  [unwired: 13 in]
      }
      frame "Macro: Exit" {
        # "Tell RT Target to ShutDown"
        # "Set Stop Global Variable to True"
        # "Exit Macro\n(This is called once, when the VI exits)"
        n131 = Unbundle By Name(w388) -> ("Core.Close Panel on Exit?"=w387:bool)
        n132 = Bundle By Name(cluster=T19 {"Command"="", "Data"=variant} ("InterProcessQueue"), "Command"="IP: ShutDown") -> (w379:T19)
        n133 = Enqueue Element(queue=w374, element=w379, error in (no error)=w377) -> (error out=w376:errorcluster)  [unwired: 1 in, 2 out]
        n134 = shared-variable ".\\Variables.lvlib\\Stop"(TRUE ("Stop"), error in=w376) -> (error out=w375:errorcluster)
        n135 = Select(t="UI: Front Panel State >> Close", s=w387, f="") -> (s? t:f=w384:string)
        n136 = call <vilib>:"Add State(s) to Queue__jki_lib_state_machine.vi"("State(s) in (\"\")"=w384, "State(s) at Back (\"\")"="Data: Cleanup\nConfig: SaveConfiguration\nStatus: Update >> Exiting Program\nExit") -> ("States Out"=w382:string)  [unwired: 13 in]
        n137 = call <vilib>:"Add State(s) to Queue__jki_lib_state_machine.vi"("State(s) in Front (\"\")"=w382, "State(s) in (\"\")"=w390) -> ("States Out"=w389:string)  [unwired: 13 in]
      }
      frame "---------- Config ----------" {
        # "Template Separator\n(You can make a copy of, or modify, this frame)"
        n138 = call <vilib>:"Add State(s) to Queue__jki_lib_state_machine.vi"("State(s) in (\"\")"=w394) -> ("States Out"=w393:string)  [unwired: 14 in]
      }
      frame "Config: LoadConfiguration" {
        # "Read \nentire\nfile"
        # "Template Separator\n(You can make a copy of, or modify, this frame)"
        n139 = call <vilib>:"Application Directory.vi"() -> ("Application Directory"=w420:path)
        n140 = Build Path(base path=w420, name or relative path=path "Config.json") -> (appended path=w418:path)
        n141 = Open/Create/Replace File(file path (use dialog)=w418, error in=w416, operation (0:open)=T21."open") -> (refnum out=w413:refnum<file>, error out=w414:errorcluster)  [unwired: 3 in, 1 out]
        n142 = Read from Binary File(8:w414, 10:-1 ("count (1)"), 11:w413) -> (0:w410:errorcluster, 2:w411:string, 3:w412:refnum<file>)  [unwired: 3 in, 1 out]
        n143 = call <vilib>:"Reformat.vi"("Pretty Print Levels"=0, "error in (no error)"=w410, "JSON"=w411) -> ("<JSON>"=w404:string)  [unwired: 5 in, 3 out]
        n144 = call "From JSON Text.vim"("Data Type and Default Value"=T20 {"RT Display Reader Loop Time [ms]"=0, "NI9205 Offset"={"NI9205 Offset"=[]}, "NI9205 Multiplier"={"NI9205 Multiplier"=[]}, "NI9208 Offset"={"NI9208 Offset"=[]}, "NI9208 Multiplier"={"NI9208 Multiplier"=[]}, "Apply Offset?"=FALSE, "Apply Multiplier?"=FALSE} ("Config Cluster"), "JSON"=w404) -> ("error out"=w405:errorcluster, "Data out"=w402:T20)  [unwired: 8 in]
        n145 = Unbundle By Name(w402) -> ("RT Display Reader Loop Time [ms]"=w401:i64, "NI9205 Offset"=w400:T6, "NI9205 Multiplier"=w399:T3, "NI9208 Offset"=w398:T2, "NI9208 Multiplier"=w397:T1, "Apply Offset?"=w396:T4, "Apply Multiplier?"=w395:T7)
        n146 = Close File(refnum=w412, error in=w410) -> (error out=w409:errorcluster)  [unwired: 1 out]
        n147 = Merge Errors(w405, w409) -> (w408:errorcluster)
        n148 = local write "NI9208 Offset"(w398) -> ()
        n149 = local write "NI9208 Multiplier"(w397) -> ()
        n150 = local write "RT Display Reader Loop Time [ms]"(w401) -> ()
        n151 = local write "NI9205 Offset"(w400) -> ()
        n152 = local write "NI9205 Multiplier"(w399) -> ()
        n153 = local write "Apply Offset?"(w396) -> ()
        n154 = local write "Apply Multiplier?"(w395) -> ()
        n155 = call <vilib>:"Add State(s) to Queue__jki_lib_state_machine.vi"("State(s) in Front (\"\")"="Config: SendGraphConfig\nStatus: Update >> Params loaded from Config file" ("State(s) in Front (\"\")"), "State(s) in (\"\")"=w423) -> ("States Out"=w422:string)  [unwired: 13 in]
      }
      frame "Config: SaveConfiguration" {
        # "Template Separator\n(You can make a copy of, or modify, this frame)"
        n156 = case shown="\"idle\", Default" w433 {
          tunnel: [w452 w456] -> w449
          tunnel: w432 -> [w455 _]
          frame "Export" {
            # "Use export folder path."
            n157 = Unbundle By Name(w455) -> ("Export Folder Path"=w454:path)
            n158 = Build Path(base path=w454, name or relative path=path "Config.json") -> (appended path=w452:path)
          }
          frame "idle", Default {
            # "Use Config file in project folder"
            n159 = call <vilib>:"Application Directory.vi"() -> ("Application Directory"=w458:path)
            n160 = Build Path(base path=w458, name or relative path=path "Config.json") -> (appended path=w456:path)
          }
        }
        n161 = local read "RT Display Reader Loop Time [ms]"() -> (w430:T5)
        n162 = local read "NI9205 Multiplier"() -> (w428:T3)
        n163 = local read "Apply Multiplier?"() -> (w424:T7)
        n164 = local read "NI9208 Multiplier"() -> (w426:T1)
        n165 = local read "Apply Offset?"() -> (w425:T4)
        n166 = local read "NI9205 Offset"() -> (w429:T6)
        n167 = local read "NI9208 Offset"() -> (w427:T2)
        n168 = Bundle(cluster=T20 {"RT Display Reader Loop Time [ms]"=0, "NI9205 Offset"={"NI9205 Offset"=[]}, "NI9205 Multiplier"={"NI9205 Multiplier"=[]}, "NI9208 Offset"={"NI9208 Offset"=[]}, "NI9208 Multiplier"={"NI9208 Multiplier"=[]}, "Apply Offset?"=FALSE, "Apply Multiplier?"=FALSE} ("output cluster"), "RT Display Reader Loop Time [ms]"=w430, "NI9205 Offset"=w429, "NI9205 Multiplier"=w428, "NI9208 Offset"=w427, "NI9208 Multiplier"=w426, "Apply Offset?"=w425, "Apply Multiplier?"=w424) -> (w435:T20)
        n169 = Open/Create/Replace File(file path (use dialog)=w449, error in=w437, operation (0:open)=T21."open or create") -> (refnum out=w442:refnum<file>, error out=w431:errorcluster)  [unwired: 3 in, 1 out]
        n170 = call "To JSON Text.vim"("error in (no error)"=w431, "Anything"=w435) -> ("error out"=w440:errorcluster, "<JSON>"=w444:string)  [unwired: 8 in]
        n171 = call <vilib>:"Reformat.vi"("Pretty Print Levels"=10, "error in (no error)"=w440, "JSON"=w444) -> ("error out"=w439:errorcluster, "<JSON>"=w441:string)  [unwired: 5 in, 2 out]
        n172 = Merge Errors(w439, w431) -> (w438:errorcluster)
        n173 = Write to Text File(file (use dialog)=w442, text=w441, error in=w438) -> (refnum out=w447:refnum<file>, error out=w446:errorcluster)  [unwired: 1 in, 1 out]
        n174 = Close File(refnum=w447, error in=w446) -> (error out=w436:errorcluster)  [unwired: 1 out]
        n175 = call <vilib>:"Add State(s) to Queue__jki_lib_state_machine.vi"("State(s) in Front (\"\")"="IP: ReadAIloopTimes\nStatus: Update >> Config File Updated\nConfig: LoadConfiguration" ("State(s) in Front (\"\")"), "State(s) in (\"\")"=w451) -> ("States Out"=w450:string)  [unwired: 13 in]
      }
      frame "Config: SendGraphConfig" {
        # "Send scaling parameters to graph to plot values correctly."
        # "Update Coord. Transform multipliers"
        n176 = local read "Apply Multiplier?"() -> (w459:T7)
        n177 = local read "Apply Offset?"() -> (w461:T4)
        n178 = case shown="False" w461 {
          tunnel: [w484 "NI9205 Offset"] -> w460
          tunnel: [w484 "NI9208 Offset"] -> w462
          frame False {
            n179 = Initialize Array(0.0 ("element"), 32 ("dimension size")) -> (w487:dbl[])
            n180 = Bundle(w487) -> (w484:cluster{dbl[]})  [unwired: 1 in]
          }
          frame True {
          }
        }
        n181 = case shown="False" w459 {
          tunnel: [w478 "NI9208 Multiplier"] -> w464
          tunnel: [w478 "NI9205 Multiplier"] -> w463
          frame False {
            n182 = Initialize Array(1.0 ("element"), 32 ("dimension size")) -> (w479:dbl[])
            n183 = Bundle(w479) -> (w478:cluster{dbl[]})  [unwired: 1 in]
          }
          frame True {
          }
        }
        n184 = Bundle By Name(cluster=T22 {"RT Display Reader Loop Time [ms]"=1000, "NI9205 Offset"={"NI9205 Offset"=[]}, "NI9205 Multiplier"={"NI9205 Multiplier"=[]}, "NI9208 Offset"={"NI9208 Offset"=[]}, "NI9208 Multiplier"={"NI9208 Multiplier"=[]}} ("GraphInfoCluster"), "RT Display Reader Loop Time [ms]"="RT Display Reader Loop Time [ms]", "NI9205 Offset"=w460, "NI9205 Multiplier"=w463, "NI9208 Offset"=w462, "NI9208 Multiplier"=w464) -> (w467:T22)
        n185 = call "GetChartParams.vi"("error in (no error)"=w470, "GraphInfoCluster"=w467, "DisplayWaveforms"=w473) -> ("error out"=w471:errorcluster, "ChartParams"=w466:T25, "DisplayWaveforms out"=w472:refnum<class "DisplayWaveforms.lvclass">)  [unwired: 6 in]
        n186 = call "SetChartParams.vi"("error in (no error)"=w471, "ChartParams"=w466, "DisplayWaveforms"=w472) -> ("error out"=w469:errorcluster)  [unwired: 7 in, 1 out]
        n187 = call <vilib>:"Add State(s) to Queue__jki_lib_state_machine.vi"("State(s) in Front (\"\")"="Status: Update >> Chart Params Updated" ("State(s) in Front (\"\")"), "State(s) in (\"\")"=w474) -> ("States Out"=w475:string)  [unwired: 13 in]
      }
      frame "---------- Status ----------" {
        # "Template Separator\n(You can make a copy of, or modify, this frame)"
        n188 = call <vilib>:"Add State(s) to Queue__jki_lib_state_machine.vi"("State(s) in (\"\")"=w493) -> ("States Out"=w492:string)  [unwired: 14 in]
      }
      frame "Status: Update" {
        # "Display first current and previous status update."
        # "Template Separator\n(You can make a copy of, or modify, this frame)"
        n189 = feedback-in #1(w494) -> ()
        n190 = feedback #1() -> (w495:string)  [unwired: 1 in]
        n191 = Concatenate Strings("Prev: " ("string"), w495, "\nCurr: " ("string"), w494) -> (→"Status":string)
        n192 = call <vilib>:"Add State(s) to Queue__jki_lib_state_machine.vi"("State(s) in (\"\")"=w502) -> ("States Out"=w501:string)  [unwired: 14 in]
      }
      frame "---------- Export ----------" {
        # "Template Separator\n(You can make a copy of, or modify, this frame)"
        n193 = call <vilib>:"Add State(s) to Queue__jki_lib_state_machine.vi"("State(s) in (\"\")"=w506) -> ("States Out"=w505:string)  [unwired: 14 in]
      }
      frame "Export: ChartData" {
        # "Template Separator\n(You can make a copy of, or modify, this frame)"
        n194 = call <vilib>:"Add State(s) to Queue__jki_lib_state_machine.vi"("State(s) in Front (\"\")"="Config: SaveConfiguration >> Export\nStatus: Update >> Charts Exported" ("State(s) in Front (\"\")"), "State(s) in (\"\")"=w511) -> ("States Out"=w510:string)  [unwired: 13 in]
      }
      frame "---------- New Category ----------" {
        # "Template Separator\n(You can make a copy of, or modify, this frame)"
        n195 = call <vilib>:"Add State(s) to Queue__jki_lib_state_machine.vi"("State(s) in (\"\")"=w515) -> ("States Out"=w514:string)  [unwired: 14 in]
      }
      frame "New Category: 1" {
        # "Your code here.\n(You can make a copy of, or modify, this frame)"
        n196 = call <vilib>:"Add State(s) to Queue__jki_lib_state_machine.vi"("State(s) in (\"\")"=w519) -> ("States Out"=w518:string)  [unwired: 14 in]
      }
      frame "New Category: 2" {
        # "Your code here.\n(You can make a copy of, or modify, this frame)"
        n197 = call <vilib>:"Add State(s) to Queue__jki_lib_state_machine.vi"("State(s) in (\"\")"=w523) -> ("States Out"=w522:string)  [unwired: 14 in]
      }
    }
  }
  n198 = call <vilib>:"Show.vi"("error in (no error)"=w26, "SMO.UI"=w25) -> ("error out"=w56:errorcluster, "SMO.UI out"=w40:refnum<class "DisplayWaveforms.lvclass">)  [unwired: 8 in]
  n199 = while {
    tunnel: [TRUE ("Stop")] -> w34
    tunnel: w28 -> [w528]
    tunnel: w21 -> [w529]
    shift-right: [w530] -> _
    shift-left: STMLoopState_enum."Initialize" ("RTmainLoopState") -> [w531]
    shift-right: [w524] -> w1
    shift-left: w26 -> [w527]
    stop <- w525 stop-if-true
    # "Host -> Target Message Sender"
    n200 = case shown="\"Run\", Default" w531 {
      tunnel: [STMLoopState_enum."Warm-up" ("RTmainLoopState") STMLoopState_enum."Run" ("RTmainLoopState") w540 STMLoopState_enum."ShutDown" ("RTmainLoopState")] -> w530
      tunnel: w529 -> [_ _ w544 _]
      tunnel: w528 -> [_ _ w545 _]
      tunnel: w527 -> [w533 w535 w543 w576]
      tunnel: [w533 w535 w541 w575] -> w524
      frame "Initialize" {
      }
      frame "Warm-up" {
      }
      frame "Run", Default {
        n201 = Preview Queue Element(queue=w545, error in (no error)=w543) -> (queue out=w539:refnum<queue>, element=w537:cluster{"Command":string, "Data":variant}, error out=w542:errorcluster)  [unwired: 1 in, 1 out]
        n202 = Unbundle By Name(w537) -> ("Command"=w538:string)
        n203 = case shown="\"IP: ReadAIloopTimes\"" w538 {
          tunnel: w544 -> [_ w553 w565 w573]
          tunnel: w542 -> [w546 w550 w558 w570]
          tunnel: [w546 w552 w560 w572] -> w541
          tunnel: [STMLoopState_enum."Run" ("RTmainLoopState") STMLoopState_enum."Run" ("RTmainLoopState") STMLoopState_enum."Run" ("RTmainLoopState") STMLoopState_enum."ShutDown" ("RTmainLoopState")] -> w540
          tunnel: w539 -> [_ w549 w557 w569]
          frame "idle", Default {
          }
          frame "IP: ReadAIloopTimes" {
            n204 = Dequeue Element(queue=w549, error in (no error)=w550) -> (error out=w548:errorcluster)  [unwired: 1 in, 3 out]
            n205 = call-poly <vilib>:"Write Message.vi"("error in"=w548, "name"="PC: ReadAIloopTimes", "connection info in"=w553) -> ("error out"=w552:errorcluster)  [unwired: 7 in, 1 out]
          }
          frame "IP: SetRTtimedLoop_dt" {
            n206 = Dequeue Element(queue=w557, error in (no error)=w558) -> (element=w556:cluster{"Command":string, "Data":variant})  [unwired: 1 in, 3 out]
            n207 = Unbundle By Name(w556) -> ("Data"=w555:variant)
            n208 = Variant To Data(type=i64 0, Variant=w555) -> (data=w564:i64, error out=w562:errorcluster)  [unwired: 1 in]
            n209 = Flatten To String(anything=w564, error in (no error)=w562) -> (data string=w567:string, error out=w561:errorcluster)  [unwired: 2 in, 1 out]
            n210 = call-poly <vilib>:"Write Message.vi"("error in"=w561, "data"=w567, "name"="PC: Set RTmain_loopTime", "connection info in"=w565) -> ("error out"=w560:errorcluster)  [unwired: 6 in, 1 out]
          }
          frame "IP: ShutDown" {
            n211 = Dequeue Element(queue=w569, error in (no error)=w570) -> (error out=w568:errorcluster)  [unwired: 1 in, 3 out]
            n212 = call-poly <vilib>:"Write Message.vi"("error in"=w568, "name"="PC: ShutDown", "connection info in"=w573) -> ("error out"=w572:errorcluster)  [unwired: 7 in, 1 out]
          }
        }
      }
      frame "ShutDown" {
        n213 = shared-variable ".\\Variables.lvlib\\Stop"(TRUE ("Stop"), error in=w576) -> (error out=w575:errorcluster)
      }
    }
    n214 = shared-variable ".\\Variables.lvlib\\Stop"() -> (w526:bool)  [unwired: 1 in, 1 out]
    n215 = Or(x=w524, y=w526) -> (x .or. y?=w525:bool)
  }
  n216 = while {
    tunnel: [TRUE ("Stop")] -> w33
    tunnel: w21 -> [w585]
    shift-right: [w584] -> _
    shift-left: STMLoopState_enum."Initialize" ("RTmainLoopState") -> [w586]
    shift-right: [w580] -> w19
    shift-left: w26 -> [w583]
    tunnel: w8 -> [w579]
    stop <- w581 stop-if-true
    # "Target -> Host Message Parser"
    n217 = case shown="\"Run\", Default" w586 {
      tunnel: w585 -> [_ _ w599 _]
      tunnel: [STMLoopState_enum."Warm-up" ("RTmainLoopState") STMLoopState_enum."Run" ("RTmainLoopState") STMLoopState_enum."Run" ("RTmainLoopState") STMLoopState_enum."ShutDown" ("RTmainLoopState")] -> w584
      tunnel: w583 -> [w588 w590 w598 w631]
      tunnel: [w588 w590 w593 w631] -> w580
      tunnel: w579 -> [_ _ w592 _]
      frame "Initialize" {
      }
      frame "Warm-up" {
      }
      frame "Run", Default {
        n218 = call-poly <vilib>:"Read Message.vi"("options"=T26 {"ignore timeout error"=TRUE, "timeout ms (1000)"=1000}, "error in"=w598, "connection info in"=w599) -> ("error out"=w596:errorcluster, "name"=w595:T14, "data string"=w594:string, "timed out?"=w597:bool)  [unwired: 2 in, 3 out]
        n219 = case shown="False" w597 {
          tunnel: w596 -> [w604 w630]
          tunnel: w595 -> [w606 _]
          tunnel: w594 -> [w605 _]
          tunnel: [w603 w630] -> w593
          tunnel: w592 -> [w602 _]
          frame False {
            n220 = case shown="\"RT: GetAIloopTimes\"" w606 {
              tunnel: w605 -> [_ w617 w625 w628]
              tunnel: w604 -> [w607 w616 w624 w629]
              tunnel: [w607 w615 w621 w629] -> w603
              tunnel: w602 -> [_ _ w620 _]
              frame "idle", Default {
              }
              frame "RT: GetAIloopTimes" {
                w610 = 1000.0 ("x")
                n221 = Unflatten From String(type=T27 {"NI 9205 loop time"=0.0, "NI 9208 loop time"=0.0} ("AI loop times [s]"), binary string=w617, error in (no error)=w616) -> (value=w613:T27, error out=w615:errorcluster)  [unwired: 2 in, 1 out]
                n222 = Unbundle By Name(w613) -> ("NI 9205 loop time"=w612:dbl, "NI 9208 loop time"=w611:dbl)
                n223 = Multiply(x=w610, y=w612) -> (x*y=w609:dbl)
                n224 = Multiply(x=w610, y=w611) -> (x*y=w608:dbl)
                n225 = local write "NI9205 loop time [ms]"(w609) -> ()
                n226 = local write "NI9208 loop time [ms]"(w608) -> ()
              }
              frame "RT: UpdateDispWaveform" {
                # "Scale Z, Th scales with multiplier before plotting \nin the Chart Process VI - see chart process VI"
                # "#TODO: How to pass display data by reference\nto the display process VI?"
                n227 = Unflatten From String(type=dbl[][] [], binary string=w625, error in (no error)=w624) -> (value=w618:dbl[][], error out=w623:errorcluster)  [unwired: 2 in, 1 out]
                n228 = Array Size(array=w618) -> (size(s)=→"# of display elements \nunpacked (row x col)":i32[])
                n229 = Generate User Event(user event=w620, event data cluster=w618, error in=w623) -> (error out=w621:errorcluster)  [unwired: 1 in, 1 out]
              }
              frame "RT: Error" {
                n230 = Concatenate Strings("RT Error: " ("string"), w628) -> (w626:string)
                n231 = local write "Status"(w626) -> ()
              }
            }
          }
          frame True {
          }
        }
      }
      frame "ShutDown" {
      }
    }
    n232 = shared-variable ".\\Variables.lvlib\\Stop"() -> (w582:bool)  [unwired: 1 in, 1 out]
    n233 = Or(x=w580, y=w582) -> (x .or. y?=w581:bool)
  }
  n234 = shared-variable ".\\Variables.lvlib\\Stop"(w35) -> ()  [unwired: 1 in, 1 out]
  n235 = Unregister For Events(event registration refnum=w37) -> (error out=w59:errorcluster)  [unwired: 1 in]
  n236 = Merge Errors(w7, w56) -> (w36:errorcluster)
  n237 = shared-variable ".\\Variables.lvlib\\Stop"(w33) -> ()  [unwired: 1 in, 1 out]
  n238 = Merge Errors(w19, w1) -> (w20:errorcluster)
  n239 = call <vilib>:"Clear Errors.vi"("error in (no error)"=w1) -> ("error out"=w2:errorcluster)  [unwired: 5 in, 1 out]
  n240 = shared-variable ".\\Variables.lvlib\\Stop"(w34) -> ()  [unwired: 1 in, 1 out]
  n241 = call <vilib>:"Destroy.vi"("error in (no error)"=w36, "SMO"=w40) -> ("error out"=w58:errorcluster)  [unwired: 9 in]
  n242 = call-poly <vilib>:"Get Connection Reference.vi"("error in"=w20, "connection info in"=w21) -> ("error out"=w24:errorcluster, "connection ID out"=w22:refnum<k5>)  [unwired: 7 in, 1 out]
  n243 = property on="Stop" class="Bool (strict)"(error in=w2, "Val(Sgnl)"=TRUE ("Value (Signaling)")) -> (error out=w5:errorcluster)  [unwired: 1 in, 1 out]
  n244 = TCP Close Connection(connection ID=w22, error in (no error)=w24) -> (error out=w23:errorcluster)  [unwired: 1 in, 1 out]
  n245 = call "Specific Error Handler"("Error to Check"=w23) -> ("error out"=w4:errorcluster)  [unwired: 11 in, 3 out]
  n246 = Merge Errors(w4, w5) -> (w3:errorcluster)
  n247 = Merge Errors(w59, w58, w3) -> (w18:errorcluster)
  n248 = call "Close Queues.vi"("error in (no error)"=w18, "FIFOs In"=w12) -> ("error out"=w17:errorcluster)  [unwired: 9 in]
  n249 = call <vilib>:"Simple Error Handler.vi"("error in (no error)"=w17) -> ()  [unwired: 4 in, 5 out]
